vi "confMedicion.vi"(8 "error in (no error)":errorcluster) -> (0 "error out":errorcluster)   [LabVIEW 2019, in "K2002_GPIB.lvlib"]
uses:
  K2002_GPIB.lvlib
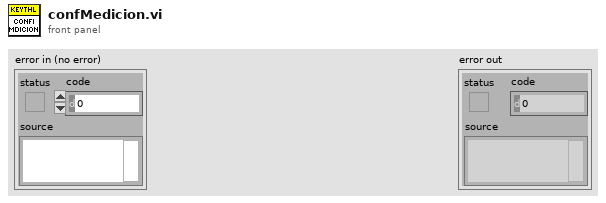
[diagram p1: front panel]
types:
  T1 = cluster{"error":bool, "code":i32, "source":string}
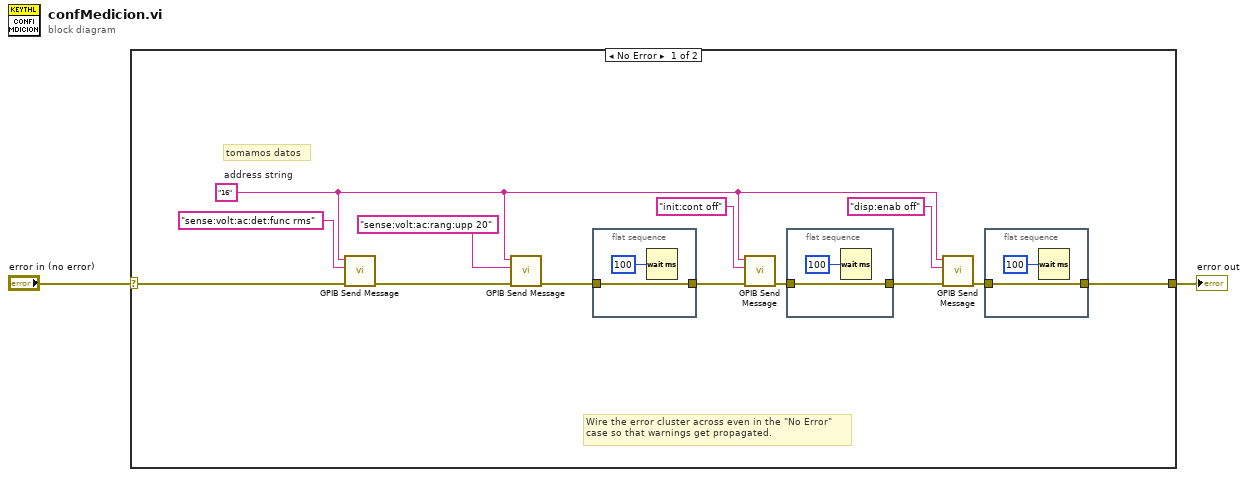
[diagram p0: block diagram]
diagram:
  n1 = case shown="No Error" "error in (no error)" {
    selector: "error in (no error)" -> [w4 w22]
    tunnel: [w3 w22] -> w1
    frame No Error {
      w5 = "16"  # address string
      # "tomamos datos"
      # "Wire the error cluster across even in the \"No Error\"\ncase so that warnings get propagated."
      n2 = call <instrlib>:"GPIB Send Message.vi"("address string"=w5, "write buffer"="sense:volt:ac:det:func rms", "error in"=w4) -> ("error out"=w12:T1)  [unwired: 4 in, 2 out]
      n3 = call <instrlib>:"GPIB Send Message.vi"("address string"=w5, "write buffer"="sense:volt:ac:rang:upp 20", "error in"=w12) -> ("error out"=w7:T1)  [unwired: 4 in, 2 out]
      n4 = flat-sequence {
        tunnel: w7 -> [w21]
        tunnel: [w21] -> w11
        frame #0 {
          n5 = Wait (ms)(milliseconds to wait=u32 100) -> ()  [unwired: 1 out]
        }
      }
      n6 = call <instrlib>:"GPIB Send Message.vi"("address string"=w5, "write buffer"="init:cont off", "error in"=w11) -> ("error out"=w10:T1)  [unwired: 4 in, 2 out]
      n7 = flat-sequence {
        tunnel: w10 -> [w19]
        tunnel: [w19] -> w9
        frame #0 {
          n8 = Wait (ms)(milliseconds to wait=u32 100) -> ()  [unwired: 1 out]
        }
      }
      n9 = call <instrlib>:"GPIB Send Message.vi"("address string"=w5, "write buffer"="disp:enab off", "error in"=w9) -> ("error out"=w8:T1)  [unwired: 4 in, 2 out]
      n10 = flat-sequence {
        tunnel: w8 -> [w17]
        tunnel: [w17] -> w3
        frame #0 {
          n11 = Wait (ms)(milliseconds to wait=u32 100) -> ()  [unwired: 1 out]
        }
      }
    }
    frame Error {
    }
  }
  "error out" <- w1
